vi "Client Test.vi"   [LabVIEW 2019, in "NW and PSD_client.lvlib" / "NW and PSD_client.lvclass"]
uses:
  NW and PSD_client.lvclass
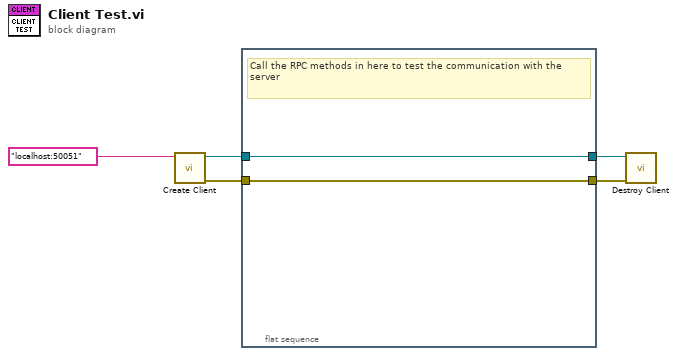
[diagram p0: block diagram]
diagram:
  n1 = call "Create Client.vi"("address"="localhost:50051") -> ("error out"=w1:errorcluster, "gRPC Client out"=w3:refnum<class "NW and PSD_client.lvclass">)  [unwired: 9 in]
  n2 = flat-sequence {
    tunnel: [w7] -> w4
    tunnel: w3 -> [w7]
    tunnel: [w6] -> w2
    tunnel: w1 -> [w6]
    frame #0 {
      # "Call the RPC methods in here to test the communication with the server"
    }
  }
  n3 = call "Destroy Client.vi"("error in (no error)"=w2, "gRPC Client in"=w4) -> ()  [unwired: 8 in, 2 out]
